vi "process frame.vi"(9 "Bytes":u8[](array[numeric]), 10 "Message Queue in":refnum<class "Delacor_lib_QMH_Message Queue.lvclass">, 11 "ASCII in":refnum<class "ASCII.lvclass">) -> (2 "Message Queue out":refnum<class "Delacor_lib_QMH_Message Queue.lvclass">, 3 "ASCII out":refnum<class "ASCII.lvclass">)   [LabVIEW 2017, in "ISA010_module.lvlib"]
uses:
  ISA010_module.lvlib
  <vilib>/Delacor/Delacor QMH/Libraries/Message Queue_class/Delacor_lib_QMH_Message Queue.lvclass
  libraries/ModBUS.lvlibp/ASCII/ASCII.lvclass
  <vilib>/Delacor/Delacor QMH/Libraries/Message Queue_class/Delacor_lib_QMH_Message Queue.lvclass/Delacor_lib_QMH_Message Queue.ctl
  <vilib>/Delacor/Delacor QMH/Libraries/Message Queue_class/Delacor_lib_QMH_Enqueue Message (Single).vi
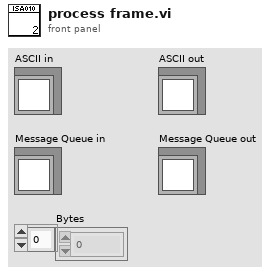
[diagram p1: front panel]
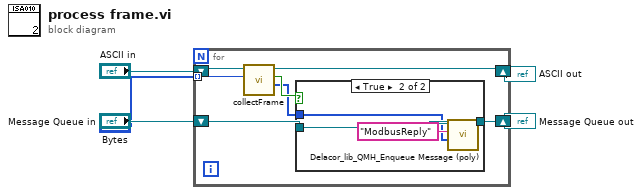
[diagram p0: block diagram]
diagram:
  n1 = for {
    tunnel: "Bytes" -> [w12] mode=indexing
    shift-right: [w10] -> w3
    shift-left: "ASCII in" -> [w11]
    shift-right: [w6] -> w5
    shift-left: "Message Queue in" -> [w7]
    n2 = call-dynamic "collectFrame.vi"("byte"=w12, "ASCII in"=w11) -> ("Data"=w8:i16[], "Finished"=w9:bool, "ASCII out"=w10:refnum<class "ASCII.lvclass">)  [unwired: 5 in, 2 out]
    n3 = case shown="True" w9 {
      tunnel: w8 -> [_ w14]
      tunnel: w7 -> [w13 w17]
      tunnel: [w13 w16] -> w6
      frame False {
      }
      frame True {
        n4 = call-poly <vilib>:"Delacor_lib_QMH_Enqueue Message (poly).vi"("Message Data"=w14, "Message"="ModbusReply", "Message Queue in"=w17) -> ("Message Queue out"=w16:refnum<class "Delacor_lib_QMH_Message Queue.lvclass">)  [unwired: 7 in, 1 out]
      }
    }
  }
  "Message Queue out" <- w5
  "ASCII out" <- w3
